vi "readAvailable.vi"(8 "error in (no error)":errorcluster, 11 "SerialCommunicator in":refnum<class "SerialCommunicator.lvclass">) -> (0 "error out":errorcluster, 2 "stringRead":string, 3 "SerialCommunicator out":refnum<class "SerialCommunicator.lvclass">)   [LabVIEW 2015, in "SerialProtocols.lvlib" / "SerialCommunicator.lvclass"]
uses:
  <userlib>/Common/SerialProtocols/SerialCommunicator/SerialCommunicator.lvclass
  <userlib>/Common/SerialProtocols/SerialCommunicator/SerialCommunicator.lvclass/SerialCommunicator.ctl
  <userlib>/Common/SerialProtocols/SerialProtocol/SerialProtocol/SerialProtocol.lvclass
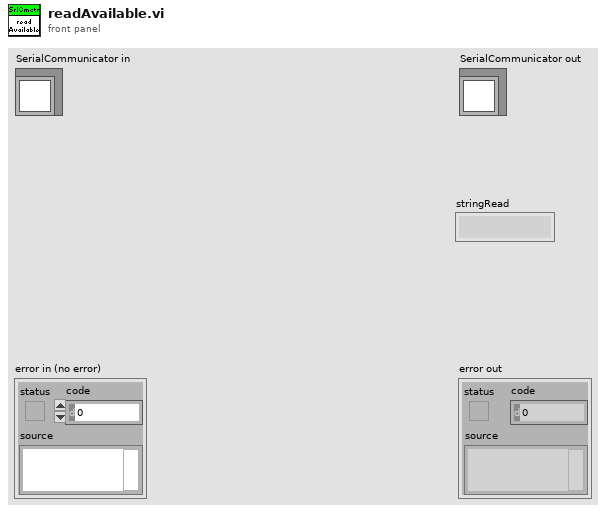
[diagram p1: front panel]
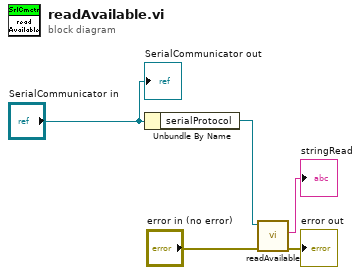
[diagram p0: block diagram]
diagram:
  n1 = Unbundle By Name("SerialCommunicator in") -> ("serialProtocol"=w4:refnum<class "SerialProtocol.lvclass">)
  n2 = call-dynamic "readAvailable.vi"("error in (no error)"="error in (no error)", "SerialProtocol in"=w4) -> ("error out"=→"error out":errorcluster, "stringRead"=→"stringRead":string)  [unwired: 7 in, 1 out]
  "SerialCommunicator out" <- "SerialCommunicator in"
